vi "Create 1.0 Servo Motor.vi"(8 "error in (no error)":errorcluster, 9 "apply offset angle from file (T)":bool=TRUE, 10 "servo ID":i32, 11 "Parallax standard servo":refnum<class "Parallax Standard Servo.lvclass">) -> (0 "error out":errorcluster, 3 "Starter Kit Servo Motor_1.0 out":refnum<class "NI_Robotics_Starter Kit Servo Motor_1.0.lvclass">)   [LabVIEW 2017, in "NI_Robotics_Starter Kit Servo Motor_1.0.lvclass"]
uses:
  <vilib>/robotics/Starter Kit/Servo Motor 1.0/NI_Robotics_Starter Kit Servo Motor_1.0.lvclass
  c:/Program Files (x86)/National Instruments/LabVIEW 2017/vi.lib/robotics/Starter Kit/Servo Motor/NI_Robotics_Starter Kit Servo Motor.lvclass
  <instrlib>/Parallax Standard Servo/HAIOL/Parallax Standard Servo.lvclass
  <vilib>/robotics/Starter Kit/Servo Motor 1.0/NI_Robotics_Starter Kit Servo Motor_1.0.lvclass/NI_Robotics_Starter Kit Servo Motor_1.0.ctl
  <vilib>/robotics/Starter Kit/Servo Motor/NI_Robotics_Starter Kit Servo Motor.lvclass/NI_Robotics_Starter Kit Servo Motor.ctl
  <vilib>/robotics/Starter Kit/Servo Motor/Apply Offset Angle.vi
  <vilib>/robotics/Starter Kit/Servo Motor/Load Offset Angle from File.vi
  <vilib>/robotics/Starter Kit/Servo Motor/NI_Robotics_Starter Kit Servo Motor.lvclass
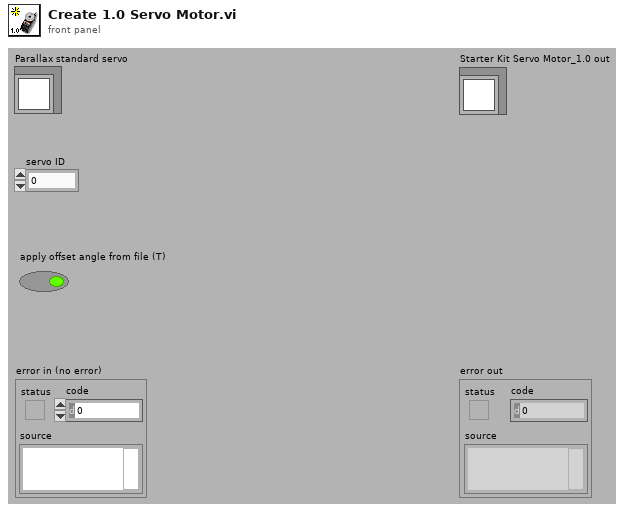
[diagram p1: front panel]
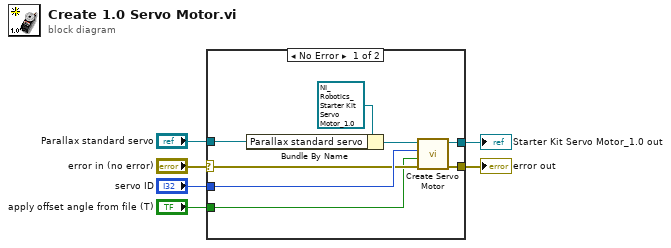
[diagram p0: block diagram]
diagram:
  n1 = case shown="No Error" "error in (no error)" {
    selector: "error in (no error)" -> [w10 w15]
    tunnel: [w9 w15] -> w5
    tunnel: "Parallax standard servo" -> [w12 _]
    tunnel: "servo ID" -> [w11 _]
    tunnel: [w8 _] -> w2
    tunnel: "apply offset angle from file (T)" -> [w7 _]
    frame No Error {
      n2 = Bundle By Name(cluster=refnum<class "NI_Robotics_Starter Kit Servo Motor_1.0.lvclass"> refnum ("Starter Kit Servo Motor_1.0 out"), "Parallax standard servo"=w12) -> (w13:refnum<class "NI_Robotics_Starter Kit Servo Motor_1.0.lvclass">)
      n3 = call <vilib>:"Create Servo Motor.vi"("error in (no error)"=w10, "apply offset angle from file (T)"=w7, "servo ID"=w11, "starter kit servo motor in"=w13) -> ("error out"=w9:errorcluster, "starter kit servo motor out"=w8:refnum<class "NI_Robotics_Starter Kit Servo Motor_1.0.lvclass">)  [unwired: 6 in]
    }
    frame Error {
    }
  }
  "error out" <- w5
  "Starter Kit Servo Motor_1.0 out" <- w2
